vi "test-quintic-spline-04.vi"() -> (3 "Test Passed":bool)   [LabVIEW 2019]
uses:
  <vilib>/Rock Robotics/WPI/ThirdParty/JAS_Junk/TrajLib/POSEwCURVATURE.ctl
  <vilib>/Rock Robotics/WPI/ThirdParty/JAS_Junk/TrajLib/POSE2D.ctl
  <vilib>/Rock Robotics/WPI/ThirdParty/JAS_Junk/TrajLib/TRANSLATION2D.ctl
  <vilib>/Rock Robotics/WPI/ThirdParty/JAS_Junk/TrajLib/ROTATION2D.ctl
  <vilib>/Rock Robotics/WPI/ThirdParty/JAS_Junk/TrajLib/Rotation2d_CreateAngle.vi
  <vilib>/Rock Robotics/WPI/ThirdParty/JAS_Junk/TrajLib/Translation2d_Create.vi
  <vilib>/Rock Robotics/WPI/ThirdParty/JAS_Junk/TrajLib/Util_CalcDist.vi
  <vilib>/Rock Robotics/WPI/ThirdParty/JAS_Junk/TrajLib/Trajectory_Library.lvlib
panel:
  out "XY Graph":cluster{dbl[], dbl[]}(graph)
  out "Numb\nWaypoints":i32
  out "All Interior \nwayPoints\nFound (True)":bool
  out "end rot = 0":dbl
  out "end y = 0":dbl
  out "end x = 0":dbl
  out "start rot = 0":dbl
  out "start y = 0":dbl
  out "start x = 0":dbl
  out "max dtheta < 0.0872":dbl
  out "max dy < 0.00127":dbl
  out "max dx  < 0.127":dbl
  out "Overall Error":errorcluster
  out "Elements":i32
  out "Create Spline Error":errorcluster
  out "SplinePoses\nWCurve":T1[](array[typedef]) {"POSE"."ROTATION"."SIN" format="%13.4f"; "POSE"."ROTATION"."COS" format="%13.4f"; "POSE"."ROTATION"."VALUE" format="%13.4f"; "POSE"."TRANSLATION"."Y" format="%14.3f"; "POSE"."TRANSLATION"."X" format="%14.3f"}
  out "Elapsed Time":dbl
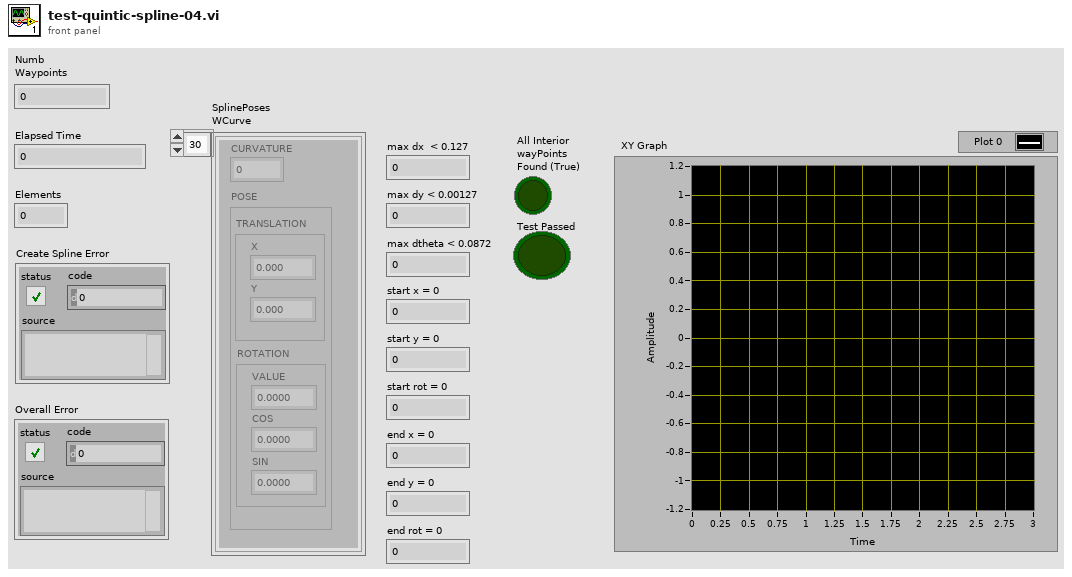
[diagram p1: front panel]
types:
  T1 = typedef "Trajectory_Library.lvlib/POSEwCURVATURE.ctl" = cluster{"CURVATURE":dbl, "POSE":T2}
  T2 = typedef "Trajectory_Library.lvlib/POSE2D.ctl" = cluster{"TRANSLATION":T3, "ROTATION":T4}
  T3 = typedef "Trajectory_Library.lvlib/TRANSLATION2D.ctl" = cluster{"X":dbl, "Y":dbl}
  T4 = typedef "Trajectory_Library.lvlib/ROTATION2D.ctl" = cluster{"VALUE":dbl, "COS":dbl, "SIN":dbl}
  T5 = typedef "Trajectory_Library.lvlib/SPLINE.ctl" = cluster{"Degree":i32, "Coefficients":T6}
  T6 = typedef "NI_Matrix.lvlib/RealMatrix.ctl" = dbl[][]
  T7 = typedef "Trajectory_Library.lvlib/TWIST2D.ctl" = cluster{"dX":dbl, "dY":dbl, "dTHETA":dbl}
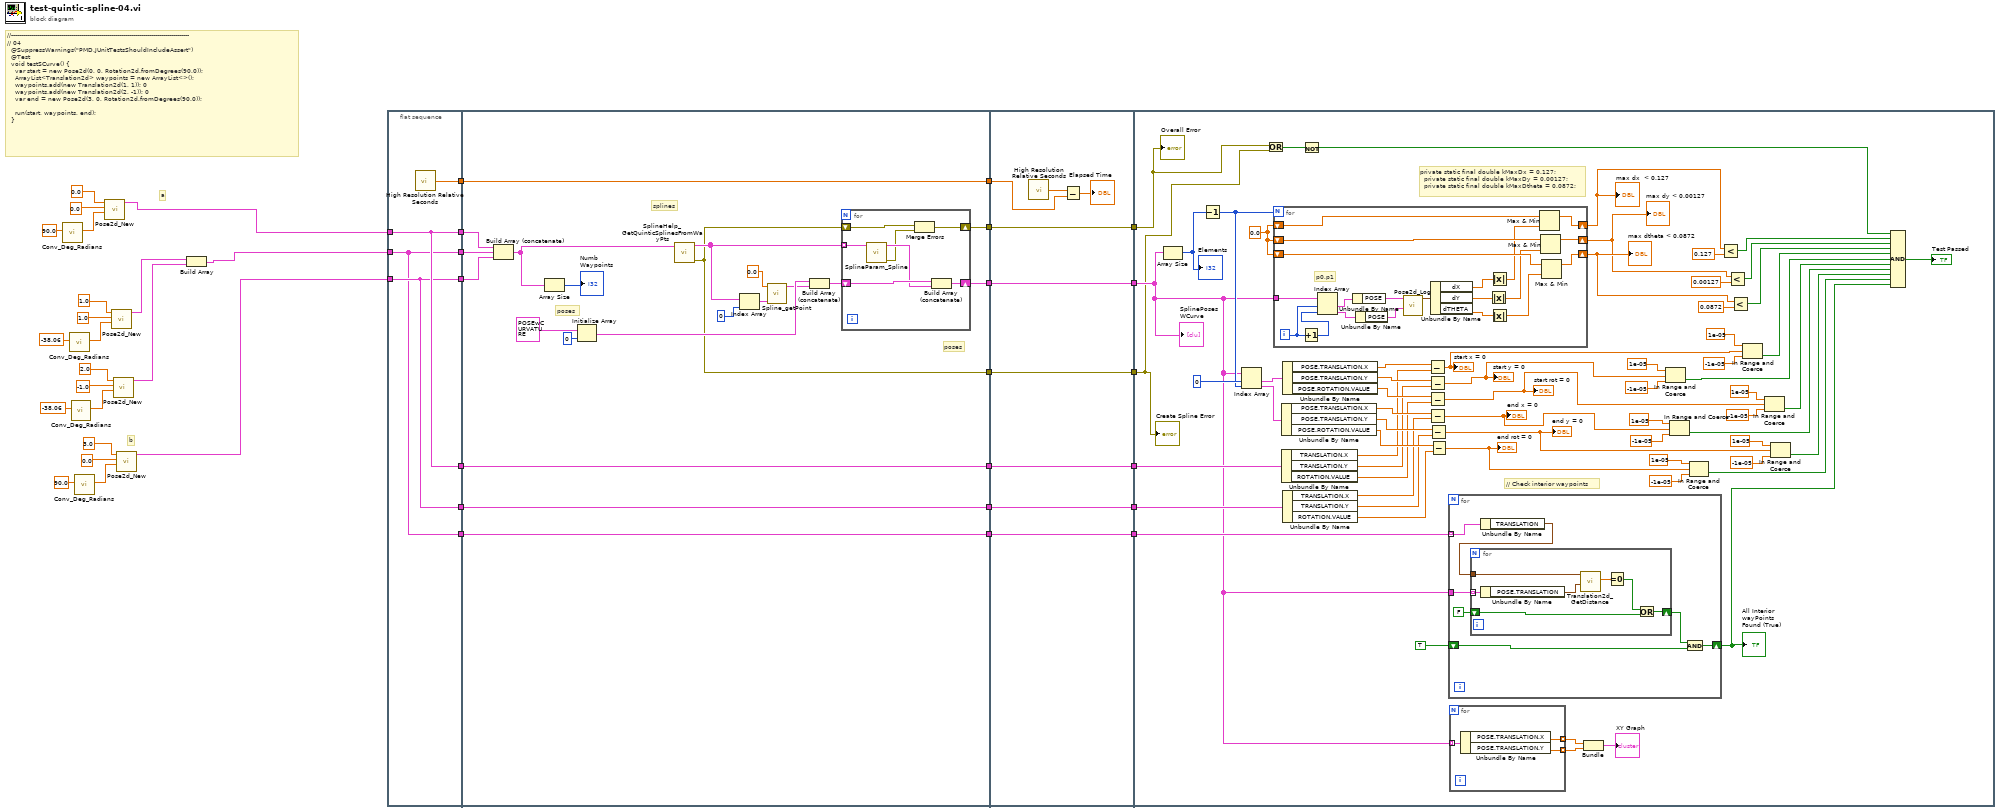
[diagram p0: block diagram]
diagram:
  # "b"
  # "a"
  # "//-----------------------------------------------------------------------------------------\n// 04\n  @SuppressWarnings(\"PMD.JUnitTestsShouldIncludeAssert\")\n  @Test\n  void testSCurve() {\n    var start = new Pose2d(0, 0, Rotation2d.fromDegrees(90.0));\n    ArrayList<Translation2d> waypoints = new ArrayList<>();\n    waypoints.add(new Translation2d(1, 1)); 0\n    waypoints.add(new Translation2d(2, -1)); 0\n    var end = new Pose2d(3, 0, Rotation2d.fromDegrees(90.0));\n\n    run(start, waypoints, end);\n  }"
  n1 = call <vilib>:"Conv_Deg_Radians.vi"("Degress"=90.0) -> ("Radians"=w16:dbl)  [unwired: 10 in]
  n2 = call <vilib>:"Conv_Deg_Radians.vi"("Degress"=-38.06) -> ("Radians"=w11:dbl)  [unwired: 10 in]
  n3 = call <vilib>:"Conv_Deg_Radians.vi"("Degress"=-38.06) -> ("Radians"=w7:dbl)  [unwired: 10 in]
  n4 = call <vilib>:"Conv_Deg_Radians.vi"("Degress"=90.0) -> ("Radians"=w19:dbl)  [unwired: 10 in]
  n5 = call <vilib>:"Pose2d_New.vi"("Heading"=w16, "Y"=0.0, "X"=0.0) -> ("out POSe"=w3:T2)  [unwired: 8 in]
  n6 = call <vilib>:"Pose2d_New.vi"("Heading"=w11, "Y"=1.0, "X"=1.0) -> ("out POSe"=w5:T2)  [unwired: 8 in]
  n7 = call <vilib>:"Pose2d_New.vi"("Heading"=w7, "Y"=-1.0, "X"=2.0) -> ("out POSe"=w4:T2)  [unwired: 8 in]
  n8 = call <vilib>:"Pose2d_New.vi"("Heading"=w19, "Y"=0.0, "X"=3.0) -> ("out POSe"=w1:T2)  [unwired: 8 in]
  n9 = Build Array(w5, w4) -> (w2:T2[])
  n10 = flat-sequence {
    tunnel: w3 -> [w44]
    tunnel: [w44] -> w41
    tunnel: w1 -> [w43]
    tunnel: [w43] -> w40
    tunnel: [w45] -> w39
    tunnel: [w44] -> w31
    tunnel: [w43] -> w28
    tunnel: [w42] -> w23
    tunnel: w2 -> [w42]
    tunnel: [w42] -> w22
    tunnel: w41 -> [w50]
    tunnel: w40 -> [w49]
    tunnel: [w66] -> w38
    tunnel: w39 -> [w66]
    tunnel: [w56] -> w37
    tunnel: [w55] -> w35
    tunnel: [w54] -> w33
    tunnel: w31 -> [w53]
    tunnel: [w53] -> w30
    tunnel: w28 -> [w52]
    tunnel: [w52] -> w27
    tunnel: [w51] -> w24
    tunnel: w23 -> [w51]
    tunnel: w22 -> [w47]
    tunnel: w38 -> [w82]
    tunnel: w37 -> [w81]
    tunnel: [w81] -> w36
    tunnel: w35 -> [w80]
    tunnel: [w80] -> w34
    tunnel: w33 -> [w79]
    tunnel: [w79] -> w32
    tunnel: w30 -> [w76]
    tunnel: [w76] -> w29
    tunnel: w27 -> [w75]
    tunnel: [w75] -> w26
    tunnel: [w74] -> w25
    tunnel: w24 -> [w74]
    tunnel: w36 -> [w123]
    tunnel: w34 -> [w111]
    tunnel: w32 -> [w110]
    tunnel: w29 -> [w145]
    tunnel: w26 -> [w144]
    tunnel: w25 -> [w127]
    frame #0 {
      n11 = call <vilib>:"High Resolution Relative Seconds.vi"() -> ("relative seconds"=w45:dbl)
    }
    frame #1 {
      # "poses"
      # "poses"
      # "splines"
      n12 = Build Array (concatenate)(w50, w47, w49) -> (w46:T2[])
      n13 = Array Size(array=w46) -> (size(s)=→"Numb\nWaypoints":i32)
      n14 = Initialize Array(T1 {"CURVATURE"=0.0, "POSE"={"TRANSLATION"={"X"=0.0, "Y"=0.0}, "ROTATION"={"VALUE"=0.0, "COS"=1.0, "SIN"=0.0}}} ("POSEwCURVATURE"), 0 ("dimension size")) -> (w60:T1[])
      n15 = call <vilib>:"SplineHelp_GetQuinticSplinesFromWayPts.vi"("WayPoints"=w46) -> ("out Error"=w55:errorcluster, "Splines"=w57:T5[])  [unwired: 9 in]
      n16 = Index Array(array=w57, index=0) -> (element=w62:T5)
      n17 = call <vilib>:"Spline_getPoint.vi"("inputSPLINE"=w62, "Time"=0.0) -> ("POSEwCURVATURE"=w59:T1)  [unwired: 9 in]
      n18 = Build Array (concatenate)(w60, w59) -> (w58:T1[])
      n19 = for {
        shift-right: [w70] -> w56
        shift-left: w58 -> [w72]
        tunnel: w57 -> [w73] mode=indexing
        shift-right: [w68] -> w54
        shift-left: w55 -> [w69]
        n20 = call <vilib>:"SplineParam_Spline.vi"("inputSPLINE"=w73) -> ("error out"=w67:errorcluster, "outputPOSEwCURVATURE"=w71:T1[])  [unwired: 9 in]
        n21 = Merge Errors(w69, w67) -> (w68:errorcluster)
        n22 = Build Array (concatenate)(w72, w71) -> (w70:T1[])
      }
    }
    frame #2 {
      n23 = call <vilib>:"High Resolution Relative Seconds.vi"() -> ("relative seconds"=w77:dbl)
      n24 = Subtract(x=w77, y=w82) -> (x-y=→"Elapsed Time":dbl)
    }
    frame #3 {
      w146 = 0.0
      # "// Check interior waypoints"
      # "private static final double kMaxDx = 0.127;\n  private static final double kMaxDy = 0.00127;\n  private static final double kMaxDtheta = 0.0872;"
      n25 = Array Size(array=w123) -> (size(s)=w147:i32)
      "Elements" <- w147
      n26 = Decrement(x=w147) -> (x-1=w142:i32)
      n27 = Index Array(array=w123, index #1=0 ("index"), index #2=w142) -> (element #1=w141:T1, element #2=w140:T1)
      n28 = Or(x=w110, y=w111) -> (x .or. y?=w112:bool)
      n29 = for {
        N: w142 -> [_]
        tunnel: w123 -> [w182]
        shift-right: [w173] -> w116
        shift-left: w146 -> [w170]
        shift-right: [w171] -> w118
        shift-left: w146 -> [w168]
        shift-right: [w172] -> w117
        shift-left: w146 -> [w169]
        i -> [w184]
        # "p0,p1"
        n30 = Increment(x=w184) -> (x+1=w183:i32)
        n31 = Index Array(array=w182, index #1=w184, index #2=w183) -> (element #1=w181:T1, element #2=w180:T1)
        n32 = Unbundle By Name(w181) -> ("POSE"=w179:T2)
        n33 = Unbundle By Name(w180) -> ("POSE"=w178:T2)
        n34 = call <vilib>:"Pose2d_Log.vi"("end POSE"=w178, "in POSE"=w179) -> ("out TWIST"=w177:T7)  [unwired: 9 in]
        n35 = Unbundle By Name(w177) -> ("dX"=w174:dbl, "dY"=w175:dbl, "dTHETA"=w176:dbl)
        n36 = Absolute Value(x=w175) -> (abs(x)=w166:dbl)
        n37 = Absolute Value(x=w174) -> (abs(x)=w167:dbl)
        n38 = Absolute Value(x=w176) -> (abs(x)=w165:dbl)
        n39 = Max & Min(x=w170, y=w167) -> (max(x,y)=w173:dbl)  [unwired: 1 out]
        n40 = Max & Min(x=w169, y=w166) -> (max(x,y)=w172:dbl)  [unwired: 1 out]
        n41 = Max & Min(x=w168, y=w165) -> (max(x,y)=w171:dbl)  [unwired: 1 out]
      }
      "max dx  < 0.127" <- w116
      "max dy < 0.00127" <- w117
      "max dtheta < 0.0872" <- w118
      n42 = Unbundle By Name(w140) -> ("POSE.TRANSLATION.X"=w136:dbl, "POSE.TRANSLATION.Y"=w135:dbl, "POSE.ROTATION.VALUE"=w134:dbl)
      n43 = Unbundle By Name(w145) -> ("TRANSLATION.X"=w133:dbl, "TRANSLATION.Y"=w132:dbl, "ROTATION.VALUE"=w131:dbl)
      n44 = Unbundle By Name(w141) -> ("POSE.TRANSLATION.X"=w139:dbl, "POSE.TRANSLATION.Y"=w138:dbl, "POSE.ROTATION.VALUE"=w137:dbl)
      n45 = Unbundle By Name(w144) -> ("TRANSLATION.X"=w130:dbl, "TRANSLATION.Y"=w129:dbl, "ROTATION.VALUE"=w128:dbl)
      n46 = Not(x=w112) -> (.not. x?=w109:bool)
      n47 = Subtract(x=w139, y=w133) -> (x-y=w105:dbl)
      "start x = 0" <- w105
      n48 = Subtract(x=w138, y=w132) -> (x-y=w84:dbl)
      "start y = 0" <- w84
      n49 = Subtract(x=w137, y=w131) -> (x-y=w88:dbl)
      "start rot = 0" <- w88
      n50 = Subtract(x=w136, y=w130) -> (x-y=w89:dbl)
      "end x = 0" <- w89
      n51 = Subtract(x=w135, y=w129) -> (x-y=w96:dbl)
      "end y = 0" <- w96
      n52 = Subtract(x=w134, y=w128) -> (x-y=w100:dbl)
      "end rot = 0" <- w100
      n53 = for {
        tunnel: w127 -> [w152] mode=indexing
        tunnel: w123 -> [w157]
        shift-right: [w156] -> w108
        shift-left: TRUE -> [w155]
        n54 = Unbundle By Name(w152) -> ("TRANSLATION"=w151:T3)
        n55 = for {
          tunnel: w157 -> [w161] mode=indexing
          shift-right: [w164] -> w153
          shift-left: FALSE -> [w163]
          tunnel: w151 -> [w162]
          n56 = Unbundle By Name(w161) -> ("POSE.TRANSLATION"=w160:T3)
          n57 = call <vilib>:"Translation2d_GetDistance.vi"("other Translation"=w160, "In Translation"=w162) -> ("Distance"=w159:dbl)  [unwired: 9 in]
          n58 = Equal To 0?(x=w159) -> (x = 0?=w158:bool)
          n59 = Or(x=w158, y=w163) -> (x .or. y?=w164:bool)
        }
        n60 = And(x=w153, y=w155) -> (x .and. y?=w156:bool)
      }
      "All Interior \nwayPoints\nFound (True)" <- w108
      n61 = for {
        tunnel: [w150] -> w125 mode=indexing
        tunnel: [w149] -> w124 mode=indexing
        tunnel: w123 -> [w148] mode=indexing
        n62 = Unbundle By Name(w148) -> ("POSE.TRANSLATION.X"=w150:dbl, "POSE.TRANSLATION.Y"=w149:dbl)
      }
      n63 = Bundle(w125, w124) -> (→"XY Graph":cluster{dbl[], dbl[]})  [unwired: 1 in]
      n64 = In Range and Coerce(upper limit=1e-05, x=w84, lower limit=-1e-05) -> (In Range?=w85:bool)  [unwired: 1 out]
      n65 = In Range and Coerce(upper limit=1e-05, x=w89, lower limit=-1e-05) -> (In Range?=w91:bool)  [unwired: 1 out]
      n66 = In Range and Coerce(upper limit=1e-05, x=w100, lower limit=-1e-05) -> (In Range?=w101:bool)  [unwired: 1 out]
      n67 = Less?(x=w116, y=0.127) -> (x < y?=w115:bool)
      n68 = Less?(x=w117, y=0.00127) -> (x < y?=w114:bool)
      n69 = Less?(x=w118, y=0.0872) -> (x < y?=w113:bool)
      n70 = In Range and Coerce(upper limit=1e-05, x=w105, lower limit=-1e-05) -> (In Range?=w104:bool)  [unwired: 1 out]
      n71 = In Range and Coerce(upper limit=1e-05, x=w88, lower limit=-1e-05) -> (In Range?=w90:bool)  [unwired: 1 out]
      n72 = In Range and Coerce(upper limit=1e-05, x=w96, lower limit=-1e-05) -> (In Range?=w97:bool)  [unwired: 1 out]
      n73 = Compound Arithmetic op=AND(w109, w115, w114, w113, w104, w85, w90, w91, w97, w101, w108) -> (→"Test Passed":bool)
      "SplinePoses\nWCurve" <- w123
      "Create Spline Error" <- w111
      "Overall Error" <- w110
    }
  }
